vi "formatPropertyList.vi"(1 "property names":string[](array[string]), 2 "property values":variant[](array[variant])) -> (0 "strings":string[][](array[string]))   [LabVIEW 2017]
uses:
  <vilib>/Utility/tdmsutil.llb/TDMSFileViewerLocalizedText.vi
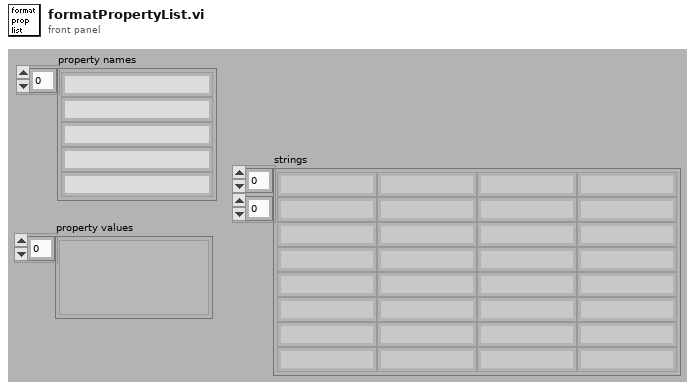
[diagram p1: front panel]
types:
  T1 = typedef "Type Enum.ctl" = enum8{"Void", "I8", "I16", "I32", "I64", "U8", "U16", "U32", "U64", "Single Float", "Double Float", "Extended Float", "Single Complex", "Double Complex", "Extended Complex", "Enum I8 NEVER", "Enum I16 NEVER", "Enum I32 NEVER", "Enum I64 NEVER", "Enum U8", "Enum U16", "Enum U32", "Enum U64", "Single Float With Unit", "Double Float With Unit", "Extended Float With Unit", "Single Complex With Unit", "Double Complex With Unit", "Extended Complex With Unit", "boolU16", "Boolean", "String", "Handle", "Path", "Picture", "C String", "Pascal String", "Tag", "SubString", "Array", "SubArray", "Cluster", "Numeric Cluster", "Variant", "LV Variant", "Measure Data (waveform)", "Refnum", "ExtData", "function", "Typedef", "Poly VI", "bad wire", "LabVIEW Class Instance"}
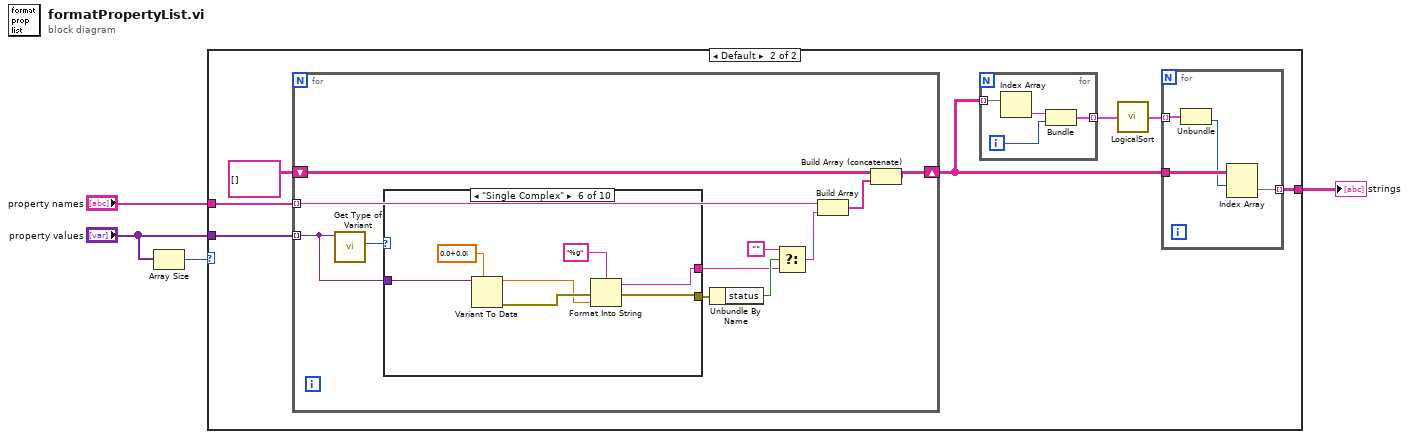
[diagram p0: block diagram]
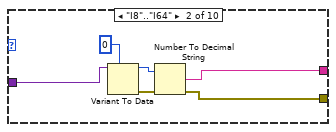
[diagram p4: hidden frame]
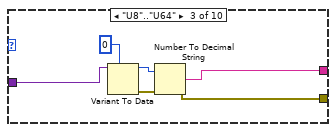
[diagram p5: hidden frame]
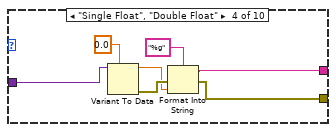
[diagram p6: hidden frame]
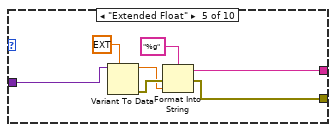
[diagram p7: hidden frame]
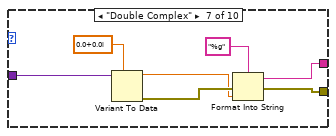
[diagram p8: hidden frame]
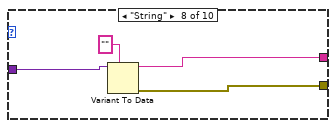
[diagram p9: hidden frame]
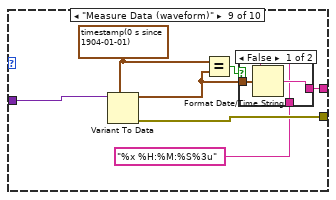
[diagram p10: hidden frame]
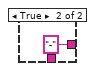
[diagram p11: hidden frame]
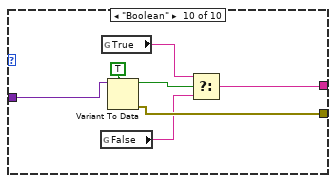
[diagram p12: hidden frame]
diagram:
  n1 = Array Size(array="property values") -> (size(s)=w2:i32)
  n2 = case shown="Default" w2 {
    tunnel: "property names" -> [_ w11]
    tunnel: "property values" -> [_ w10]
    tunnel: [_ w7] -> w1
    frame 0 {
    }
    frame Default {
      n3 = for {
        tunnel: w10 -> [w30] mode=indexing
        tunnel: w11 -> [w27] mode=indexing
        shift-right: [w28] -> w6
        shift-left: string[][] [] -> [w29]
        n4 = call <vilib>:"Get Type of Variant.vi"("Data In"=w30) -> ("Type Enum"=w26:T1)  [unwired: 9 in, 1 out]
        n5 = case shown="\"Single Complex\"" w26 {
          tunnel: w30 -> [_ w35 w40 w47 w54 w61 w68 w72 w79 w90]
          tunnel: [_ w32 w37 w44 w50 w57 w65 w70 w78 w89] -> w25
          tunnel: [_ w31 w36 w43 w49 w58 w64 w69 w77 w86] -> w23
          frame "Void", Default {
          }
          frame "I8".."I64" {
            n6 = Variant To Data(type=i64 0 ("offset (0)"), Variant=w35) -> (data=w33:i64, error out=w32:errorcluster)  [unwired: 1 in]
            n7 = Number To Decimal String(number=w33) -> (decimal integer string=w31:string)  [unwired: 1 in]
          }
          frame "U8".."U64" {
            n8 = Variant To Data(type=u64 0 ("offset (0)"), Variant=w40) -> (data=w38:u64, error out=w37:errorcluster)  [unwired: 1 in]
            n9 = Number To Decimal String(number=w38) -> (decimal integer string=w36:string)  [unwired: 1 in]
          }
          frame "Single Float", "Double Float" {
            n10 = Variant To Data(type=0.0 ("offset (0)"), Variant=w47) -> (data=w41:dbl, error out=w45:errorcluster)  [unwired: 1 in]
            n11 = Format Into String(format string="%g", error in=w45, w41) -> (resulting string=w43:string, error out=w44:errorcluster)  [unwired: 1 in]
          }
          frame "Extended Float" {
            n12 = Variant To Data(type=ext 0.0 ("offset (0)"), Variant=w54) -> (data=w48:ext, error out=w51:errorcluster)  [unwired: 1 in]
            n13 = Format Into String(format string="%g", error in=w51, w48) -> (resulting string=w49:string, error out=w50:errorcluster)  [unwired: 1 in]
          }
          frame "Single Complex" {
            n14 = Variant To Data(type=csg 0.0+0.0i, Variant=w61) -> (data=w56:csg, error out=w59:errorcluster)  [unwired: 1 in]
            n15 = Format Into String(format string="%g", error in=w59, w56) -> (resulting string=w58:string, error out=w57:errorcluster)  [unwired: 1 in]
          }
          frame "Double Complex" {
            n16 = Variant To Data(type=cdb 0.0+0.0i, Variant=w68) -> (data=w63:cdb, error out=w66:errorcluster)  [unwired: 1 in]
            n17 = Format Into String(format string="%g", error in=w66, w63) -> (resulting string=w64:string, error out=w65:errorcluster)  [unwired: 1 in]
          }
          frame "String" {
            n18 = Variant To Data(type="" ("offset (0)"), Variant=w72) -> (data=w69:string, error out=w70:errorcluster)  [unwired: 1 in]
          }
          frame "Measure Data (waveform)" {
            w76 = timestamp(0 s since 1904-01-01) ("offset (0)")
            n19 = Variant To Data(type=w76, Variant=w79) -> (data=w75:timestamp, error out=w78:errorcluster)  [unwired: 1 in]
            n20 = Equal?(x=w76, y=w75) -> (x = y?=w74:bool)
            n21 = case shown="False" w74 {
              tunnel: w75 -> [w82 _]
              tunnel: [w81 "-" ("date/time string")] -> w77
              tunnel: "%x %H:%M:%S%3u" ("time format string (%c)") -> [w80 _]
              frame False {
                n22 = Format Date/Time String(time format string (%c)=w80, seconds (now)=w82) -> (date/time string=w81:string)  [unwired: 1 in]
              }
              frame True {
              }
            }
          }
          frame "Boolean" {
            n23 = global read "TDMSFileViewerLocalizedText.vi" "False"() -> (w85:string)
            n24 = global read "TDMSFileViewerLocalizedText.vi" "True"() -> (w84:string)
            n25 = Variant To Data(type=TRUE, Variant=w90) -> (data=w87:bool, error out=w89:errorcluster)  [unwired: 1 in]
            n26 = Select(t=w84, s=w87, f=w85) -> (s? t:f=w86:string)
          }
        }
        n27 = Unbundle By Name(w25) -> ("status"=w24:bool)
        n28 = Select(t="", s=w24, f=w23) -> (s? t:f=w21:string)
        n29 = Build Array(w27, w21) -> (w20:string[])
        n30 = Build Array (concatenate)(w29, w20) -> (w28:string[][])
      }
      n31 = for {
        tunnel: w6 -> [w15] mode=indexing
        tunnel: [w12] -> w5 mode=indexing
        i -> [w13]
        n32 = Index Array(array=w15) -> (element=w14:string)  [unwired: 1 in]
        n33 = Bundle("date/time string"=w14, w13) -> (w12:cluster{"date/time string":string, i32})  [unwired: 1 in]
      }
      n34 = call <vilib>:"LogicalSort.vi"("Input Array"=w5) -> ("Sorted Array"=w8:cluster{"date/time string":string, i32}[])  [unwired: 8 in]
      n35 = for {
        tunnel: w8 -> [w18] mode=indexing
        tunnel: w6 -> [w19]
        tunnel: [w16] -> w7 mode=indexing
        n36 = Unbundle(w18) -> (w17:i32)  [unwired: 1 out]
        n37 = Index Array(array=w19, index (row)=w17) -> (element=w16:string[])  [unwired: 1 in]
      }
    }
  }
  "strings" <- w1
